vi "terminate.vi"(8 "error in (no error)":errorcluster, 11 "ImageAssemblerRK110612Spiral in":refnum<class "ImageAssemblerRK110612Spiral.lvclass">) -> (0 "error out":errorcluster, 3 "ImageAssemblerRK110612Spiral out":refnum<class "ImageAssemblerRK110612Spiral.lvclass">)   [LabVIEW 2010, in "ImageAssemblerRK110612Spiral.lvclass"]
uses:
  ImageAssemblerRK110612Spiral.lvclass
  ImageAssemblerDL090211Scaffold/ImageAssemblerDL090211Scaffold/ImageAssemblerDL090211Scaffold.lvclass
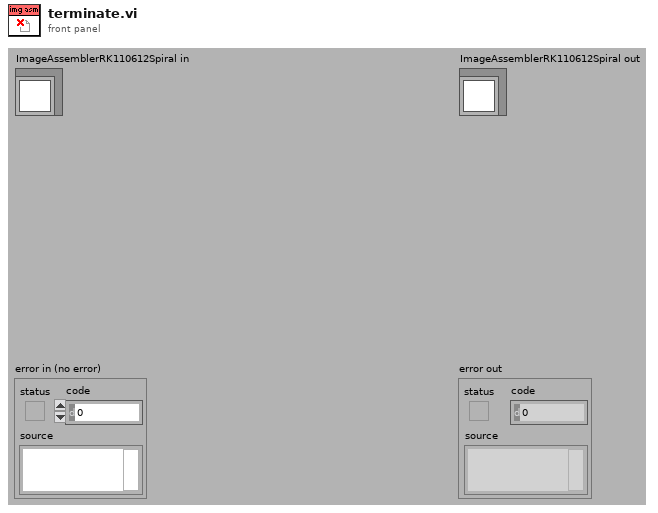
[diagram p1: front panel]
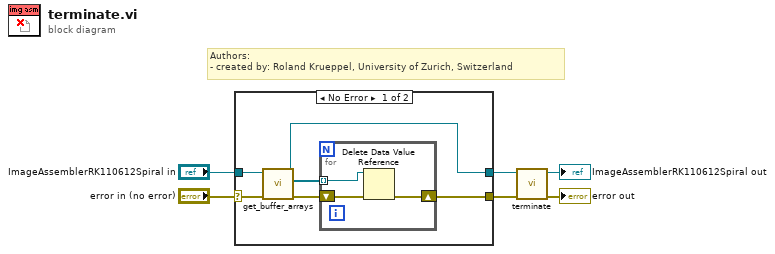
[diagram p0: block diagram]
diagram:
  # "Authors: \n- created by: Roland Krueppel, University of Zurich, Switzerland"
  n1 = case shown="No Error" "error in (no error)" {
    selector: "error in (no error)" -> [w11 w17]
    tunnel: [w7 w17] -> w3
    tunnel: [w8 w16] -> w2
    tunnel: "ImageAssemblerRK110612Spiral in" -> [w12 w16]
    frame No Error {
      n2 = call-dynamic "get_buffer_arrays.vi"("error in (no error)"=w11, "ImageAssemblerRK110612Spiral in"=w12) -> ("error out"=w10:errorcluster, "Buffer arrays"=w9:refnum<data-value>[], "ImageAssemblerRK110612Spiral out"=w8:refnum<class "ImageAssemblerRK110612Spiral.lvclass">)  [unwired: 7 in]
      n3 = for {
        shift-right: [w15] -> w7
        shift-left: w10 -> [w14]
        tunnel: w9 -> [w13] mode=indexing
        n4 = Delete Data Value Reference(data value reference=w13, error in=w14) -> (error out=w15:errorcluster)  [unwired: 1 out]
      }
    }
    frame Error {
    }
  }
  n5 = call-parent "terminate.vi"("error in (no error)"=w3, "DL090211ImageAssemblerScaffold in"=w2) -> ("error out"=→"error out":errorcluster, "DL090211ImageAssemblerScaffold out"=→"ImageAssemblerRK110612Spiral out":refnum<class "ImageAssemblerRK110612Spiral.lvclass">)  [unwired: 8 in]
